vi "Open.vi"(8 "error in (no error)":errorcluster, 11 "PDFPath":path) -> (0 "error out":errorcluster)   [LabVIEW 2019, in "Tools.lvlib"]
uses:
  Tools.lvlib
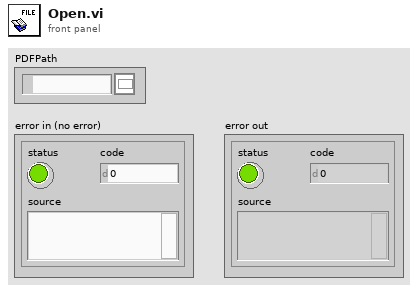
[diagram p1: front panel]
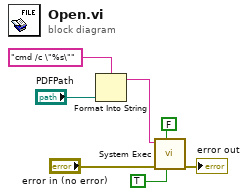
[diagram p0: block diagram]
diagram:
  n1 = Format Into String(format string="cmd /c \"%s\"", "PDFPath") -> (resulting string=w6:string)  [unwired: 2 in, 1 out]
  n2 = call <vilib>:"System Exec.vi"("run minimized? (F)"=TRUE, "wait until completion? (T)"=FALSE, "error in (no error)"="error in (no error)", "command line"=w6) -> ("error out"=→"error out":errorcluster)  [unwired: 4 in, 3 out]
